vi "Arduino to LabVIEW Communication Module.vi"() -> ()   [LabVIEW 2018]
uses:
  TypeDeclarations/GEVE Ventilator Monitoring Data.ctl
  <vilib>/Instr/_visa.llb/VISA Configure Serial Port (Instr).vi
panel:
  out "GEVE Ventilator Monitoring Data":T1
  out "loop time (ms)":u32
  out "Waveform Chart":u32(graph)
  out "read buffer data byte array":u8[](array[numeric]) format="%02x"
  in  "baud rate (9600)":u32=9600
  out "Communication Timeout?":bool
  in  "VISA resource name":refnum<visa-resource-name>="COM7"
  out "return count read":u32
  out "read buffer":string
  in  "Stop":bool
  out "Iterations":i32
  # "DEBUG AREA"
  # "iterations"
  # "poti"
  # "pressure"
  # "alarm"
  # "EOL"
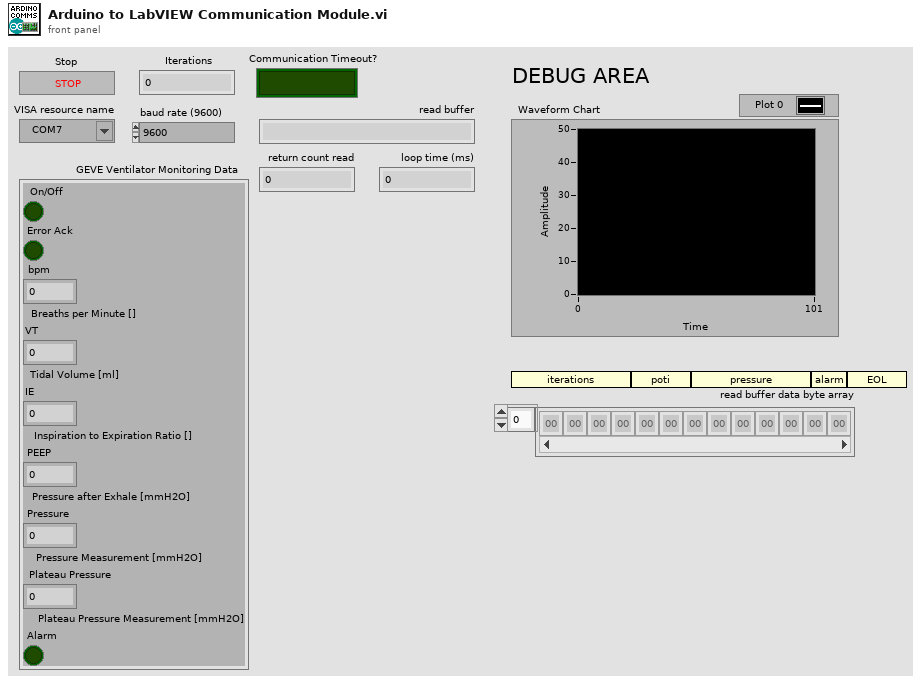
[diagram p1: front panel]
types:
  T1 = typedef "GEVE Ventilator Monitoring Data.ctl" = cluster{"On/Off":bool, "Error Ack":bool, "bpm":dbl, "VT":dbl, "IE":dbl, "PEEP":dbl, "Pressure":dbl, "Plateau Pressure":dbl, "Alarm":bool}
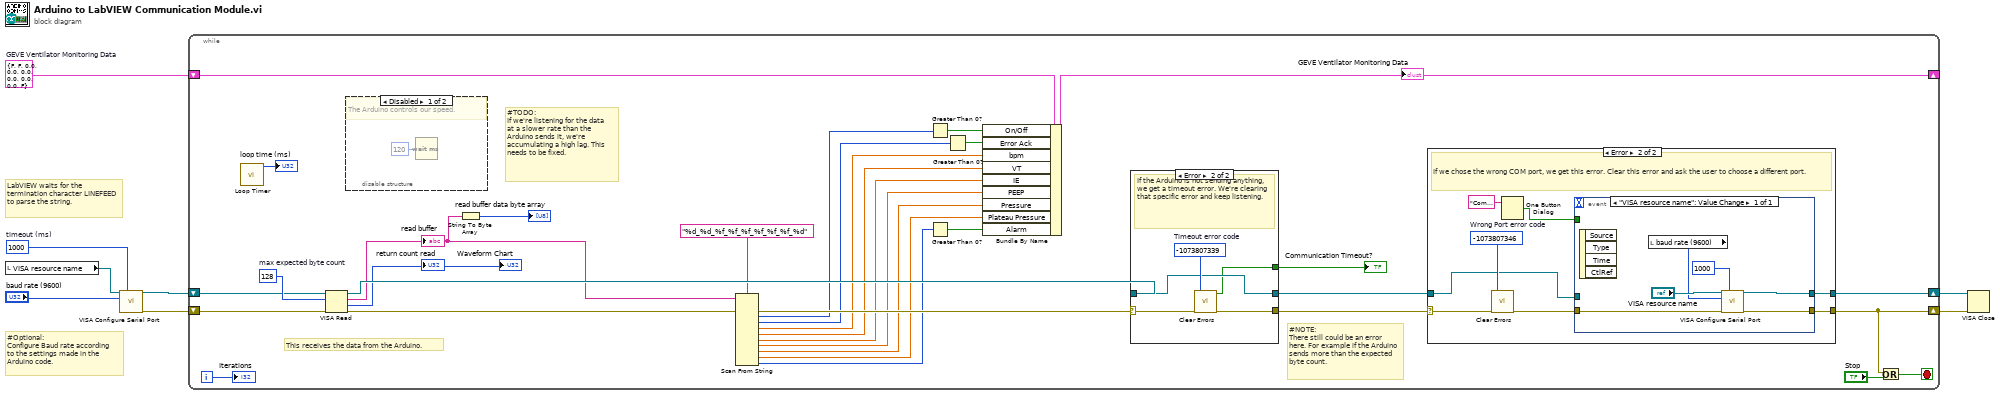
[diagram p0: block diagram]
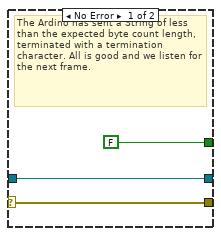
[diagram p4: hidden frame]
diagram:
  w2 = T1 {"On/Off"=FALSE, "Error Ack"=FALSE, "bpm"=0.0, "VT"=0.0, "IE"=0.0, "PEEP"=0.0, "Pressure"=0.0, "Plateau Pressure"=0.0, "Alarm"=FALSE}  # GEVE Ventilator Monitoring Data
  w4 = u32 1000  # timeout (ms)
  # "#Optional:\nConfigure Baud rate according to the settings made in the Arduino code."
  # "LabVIEW waits for the termination character LINEFEED to parse the string."
  n1 = local read "VISA resource name"() -> (w1:refnum<visa-resource-name>)
  n2 = call-poly "VISA Configure Serial Port"("VISA resource name"=w1, "timeout (10sec)"=w4, "baud rate (9600)"="baud rate (9600)") -> ("VISA resource name out"=w8:refnum<visa-resource-name>, "error out"=w6:errorcluster)  [unwired: 11 in]
  n3 = while {
    shift-right: [w10] -> w7
    shift-left: w8 -> [w30]
    shift-right: [w12] -> w5
    shift-left: w6 -> [w29]
    shift-right: [w25] -> _
    shift-left: w2 -> [w26]
    i -> [w41]
    stop <- w39 stop-if-true
    w38 = u32 128  # max expected byte count
    # "#TODO:\nIf we're listening for the data at a slower rate than the Arduino sends it, we're accumulating a high lag. This needs to be fixed."
    # "This receives the data from the Arduino."
    # "#NOTE:\nThere still could be an error here. For example if the Arduino sends more than the expected byte count."
    n4 = call "Loop Timer.vi"() -> ("loop time (ms)"=→"loop time (ms)":u32)  [unwired: 11 in]
    n5 = VISA Read(VISA resource name=w30, byte count=w38, error in (no error)=w29) -> (VISA resource name out=w37:refnum<visa-resource-name>, read buffer=w32:string, return count=→"return count read" →"Waveform Chart":u32, error out=w31:errorcluster)
    "read buffer" <- w32
    n6 = disable-structure shown="Disabled" {
      frame Disabled {
        # "The Arduino controls our speed."
        n7 = Wait (ms)(milliseconds to wait=u32 120) -> ()  [unwired: 1 out]
      }
      frame Enabled {
      }
    }
    n8 = String To Byte Array(string=w32) -> (unsigned byte array=→"read buffer data byte array":u8[])
    n9 = Scan From String(format string="%d_%d_%f_%f_%f_%f_%f_%f_%d", input string=w32, error in=w31) -> (error out=w35:errorcluster, output 1=w23:i32, output 2=w22:i32, output 3=w27:dbl, output 4=w14:dbl, output 5=w15:dbl, output 6=w16:dbl, output 7=w17:dbl, output 8=w18:dbl, output 9=w24:i32)  [unwired: 10 in, 2 out]
    n10 = Greater Than 0?(x=w23) -> (x > 0?=w21:bool)
    n11 = Greater Than 0?(x=w24) -> (x > 0?=w19:bool)
    n12 = Greater Than 0?(x=w22) -> (x > 0?=w20:bool)
    n13 = Bundle By Name(cluster=w26, "On/Off"=w21, "Error Ack"=w20, "bpm"=w27, "VT"=w14, "IE"=w15, "PEEP"=w16, "Pressure"=w17, "Plateau Pressure"=w18, "Alarm"=w19) -> (w25:T1)
    "GEVE Ventilator Monitoring Data" <- w25
    n14 = case shown="Error" w35 {
      selector: w35 -> [w61 w66]
      tunnel: [w61 w64] -> w13
      tunnel: [w60 w63] -> w11
      tunnel: w37 -> [w60 w63]
      tunnel: [FALSE ("specific error cleared?") w62] -> w36
      frame No Error {
        # "The Ardino has sent a String of less than the expected byte count length, terminated with a termination character. All is good and we listen for the next frame."
      }
      frame Error {
        w65 = -1073807339  # Timeout error code
        # "If the Arduino is not sending anything, we get a timeout error. We're clearing that specific error and keep listening."
        n15 = call <vilib>:"Clear Errors.vi"("error in (no error)"=w66, "specific error code to clear (0: all)"=w65) -> ("error out"=w64:errorcluster, "specific error cleared?"=w62:bool)  [unwired: 4 in]
      }
    }
    "Communication Timeout?" <- w36
    n16 = case shown="Error" w13 {
      selector: w13 -> [w43 w51]
      tunnel: [w43 w49] -> w12
      tunnel: [w42 w47] -> w10
      tunnel: w11 -> [w42 w46]
      frame No Error {
      }
      frame Error {
        w50 = -1073807346  # Wrong Port error code
        # "If we chose the wrong COM port, we get this error. Clear this error and ask the user to choose a different port."
        n17 = call <vilib>:"Clear Errors.vi"("error in (no error)"=w51, "specific error code to clear (0: all)"=w50) -> ("error out"=w48:errorcluster)  [unwired: 4 in, 1 out]
        n18 = One Button Dialog(message="Communication Error.\nPlease select the COM port of the GEVE Arduino.") -> (true=w44:bool)  [unwired: 1 in]
        n19 = event shown="[0] \"VISA resource name\": Value Change" {
          selector: _ -> [_]
          dyn-events: _ -> [_]
          timeout: _ -> [_]
          tunnel: [w56] -> w49
          tunnel: w48 -> [w57]
          tunnel: [w54] -> w47
          tunnel: w46 -> [_]
          tunnel: w44 -> [_]
          event "VISA resource name": Value Change {
            n20 = event-data() -> ()  [unwired: 1 in, 4 out]
            n21 = local read "baud rate (9600)"() -> (w52:u32)
            n22 = call-poly "VISA Configure Serial Port"("VISA resource name"="VISA resource name", "timeout (10sec)"=u32 1000, "baud rate (9600)"=w52, "error in (no error)"=w57) -> ("VISA resource name out"=w54:refnum<visa-resource-name>, "error out"=w56:errorcluster)  [unwired: 10 in]
          }
        }
      }
    }
    n23 = Or(x=w12, y="Stop") -> (x .or. y?=w39:bool)
    "Iterations" <- w41
  }
  n24 = VISA Close(VISA resource name=w7, error in (no error)=w5) -> ()  [unwired: 1 out]
